vi "VH4TM.vi"(10 "M":dbl, 11 "T":dbl[unit]) -> (1 "S":dbl[unit], 2 "V":dbl[unit], 3 "H":dbl[unit])   [LabVIEW 2011]
panel:
  in  "file path (use dialog)":path=path "C:/Users/lsv/Documents/Sys/AI-04/Датчик швидкості/VI/STOIL.FOR"
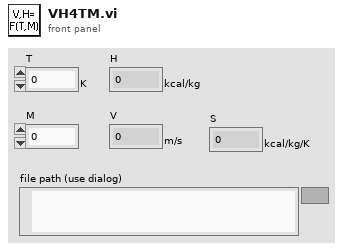
[diagram p1: front panel]
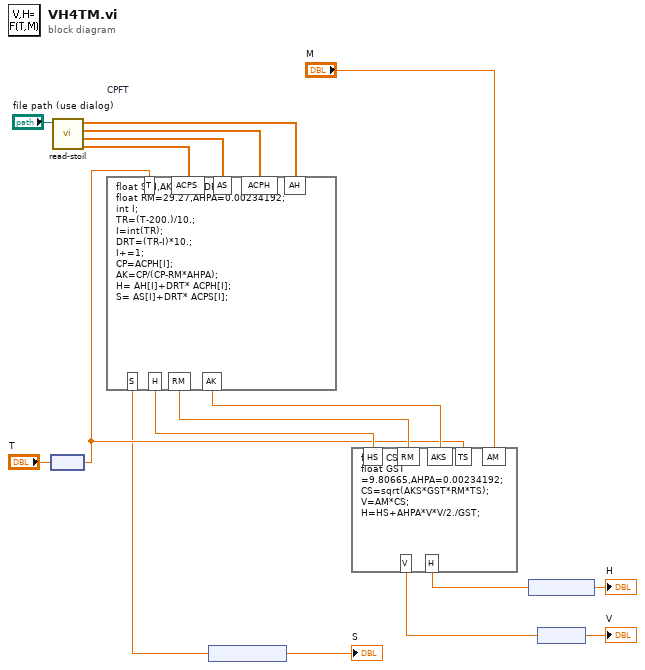
[diagram p0: block diagram]
diagram:
  n1 = node("T") -> (w6:dbl)
  n2 = call "read-stoil.vi"("file path (use dialog)"="file path (use dialog)") -> ("ACPS"=w10:dbl[], "AS"=w9:dbl[], "ACPH"=w8:dbl[], "AH"=w7:dbl[])  [unwired: 7 in]
  n3 = formula code="float S,H,AK,CP,TR,DRT;\nfloat RM=29.27,AHPA=0.00234192;\nint I;\nTR=(T-200.)/10.;\nI=int(TR); \nDRT=(TR-I)*10.;\nI+=1;\nCP=ACPH[I];\nAK=CP/(CP-RM*AHPA);\nH= AH[I]+DRT* ACPH[I];\nS= AS[I]+DRT* ACPS[I];" "CPFT"("T"=w6, "AH"=w7, "ACPH"=w8, "AS"=w9, "ACPS"=w10) -> ("S"=w3:dbl, "AK"=w11:dbl, "RM"=w12:dbl, "H"=w15:dbl)
  n4 = node(w3) -> (→"S":dbl[unit])
  n5 = formula code="float CS,V,H;\nfloat GST =9.80665,AHPA=0.00234192;\nCS=sqrt(AKS*GST*RM*TS);\nV=AM*CS;\nH=HS+AHPA*V*V/2./GST;"("AKS"=w11, "RM"=w12, "TS"=w6, "AM"="M", "HS"=w15) -> ("V"=w17:dbl, "H"=w16:dbl)
  n6 = node(w16) -> (→"H":dbl[unit])
  n7 = node(w17) -> (→"V":dbl[unit])
